vi "Add Thread Configuration.vi"(8 "error in":errorcluster, 10 "configuration":T14, 11 "thread":T1={"core"={"processor"=-2, "priority offset"=0}, "component settings"=[], "transfer groups"=[]}) -> (0 "error out":errorcluster, 3 "thread out":T1={"core"={"processor"=-2, "priority offset"=0}, "component settings"=[], "transfer groups"=[]})   [LabVIEW 2020, in "DSF UDP Configuration API.lvlib"]
uses:
  DSF UDP Configuration API.lvlib
  Built/Plugins/Windows/Components/UDP.lvlibp/Configuration/Thread/Thread Settings.ctl
  <vilib>/addons/VeriStand Custom Device Scripting APIs/Data Sharing Framework/DSF Core.lvlibp/Typedefs/DSF Engine Plugin Thread Configuration.ctl
  <vilib>/addons/VeriStand Custom Device Scripting APIs/Data Sharing Framework/DSF Core.lvlibp/Typedefs/Core Thread Configuration.ctl
  <vilib>/addons/VeriStand Custom Device Scripting APIs/Data Sharing Framework/DSF Core.lvlibp/Typedefs/DSF Settings Info.ctl
  <vilib>/addons/VeriStand Custom Device Scripting APIs/Data Sharing Framework/DSF Core.lvlibp/Typedefs/DSF Engine Transfer Group Configuration.ctl
  <vilib>/addons/VeriStand Custom Device Scripting APIs/Data Sharing Framework/DSF Core.lvlibp/Typedefs/Core Group Configuration.ctl
  <vilib>/addons/VeriStand Custom Device Scripting APIs/Data Sharing Framework/DSF Core.lvlibp/Typedefs/DSF Direction.ctl
  <vilib>/addons/VeriStand Custom Device Scripting APIs/Data Sharing Framework/DSF Core.lvlibp/Typedefs/DSF Timing Info.ctl
  <vilib>/addons/VeriStand Custom Device Scripting APIs/Data Sharing Framework/DSF Core.lvlibp/Typedefs/DSF Timeout Behavior.ctl
  <vilib>/addons/VeriStand Custom Device Scripting APIs/Data Sharing Framework/DSF Core.lvlibp/Typedefs/DSF Engine Transfer Configuration.ctl
  <vilib>/addons/VeriStand Custom Device Scripting APIs/Data Sharing Framework/DSF Core.lvlibp/Typedefs/Core Transfer Configuration.ctl
  <vilib>/addons/VeriStand Custom Device Scripting APIs/Data Sharing Framework/DSF Core.lvlibp/Typedefs/DSF Engine Channel Configuration.ctl
  <vilib>/addons/VeriStand Custom Device Scripting APIs/Data Sharing Framework/DSF Core.lvlibp/Typedefs/Core Channel Configuration.ctl
  <vilib>/addons/VeriStand Custom Device Scripting APIs/Data Sharing Framework/DSF Core.lvlibp/Typedefs/DSF Data Type.ctl
  fab8a0ae-df1d-4f1f-ba96-0da676de6823.vi
  <vilib>/addons/VeriStand Custom Device Scripting APIs/Data Sharing Framework/DSF Core.lvlibp
  Built/Plugins/Windows/Components/UDP.lvlibp/Configuration/Thread/UDP Thread Configuration.lvclass
  <vilib>/addons/VeriStand Custom Device Scripting APIs/Data Sharing Framework/DSF Core.lvlibp/Classes/Configuration/Core/Thread/Thread Configuration.lvclass
  <vilib>/addons/VeriStand Custom Device Scripting APIs/Data Sharing Framework/DSF Core.lvlibp/Classes/Configuration/Core/Group/Group Configuration.lvclass
  <vilib>/addons/VeriStand Custom Device Scripting APIs/Data Sharing Framework/DSF Core.lvlibp/Classes/Configuration/Core/Transfer/Transfer Configuration.lvclass
  <vilib>/addons/VeriStand Custom Device Scripting APIs/Data Sharing Framework/DSF Core.lvlibp/Classes/Configuration/Core/Channel/Channel Configuration.lvclass
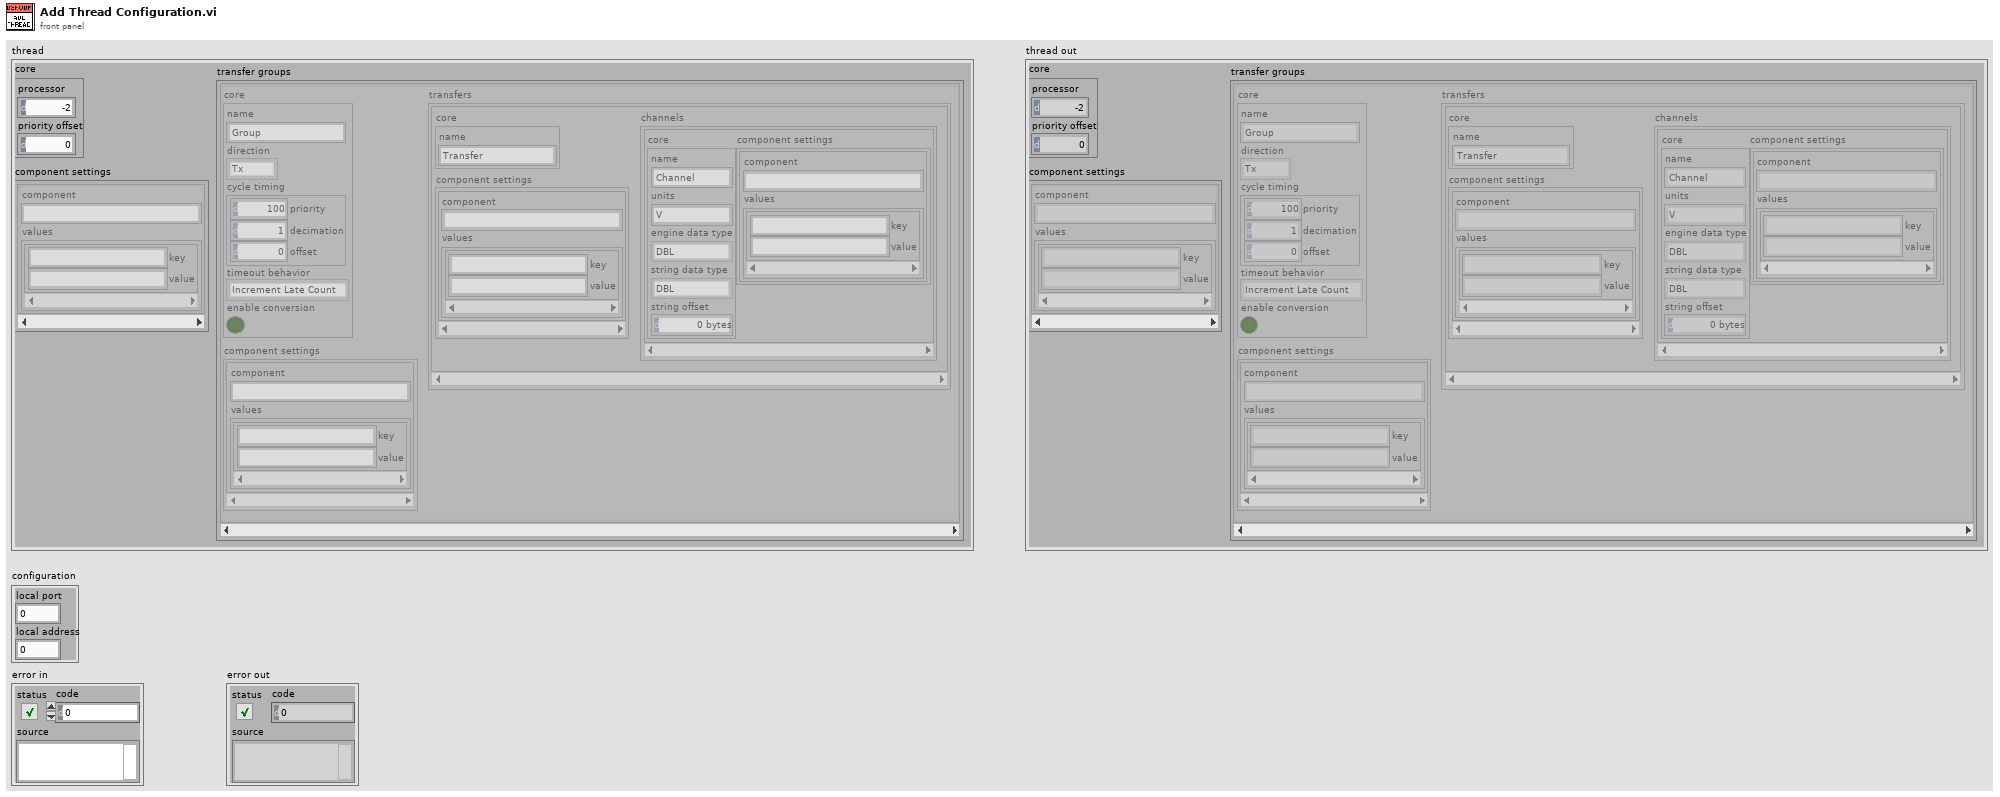
[diagram p1: front panel]
types:
  T1 = typedef "DSF Core.lvlibp/DSF Engine Plugin Thread Configuration.ctl" = cluster{"core":T2, "component settings":T3[], "transfer groups":T4[]}
  T2 = typedef "DSF Core.lvlibp/Thread Configuration.lvclass/Core Thread Configuration.ctl" = cluster{"processor":i32, "priority offset":i16}
  T3 = typedef "DSF Core.lvlibp/DSF Settings Info.ctl" = cluster{"component":string, "values":cluster{"key":string, "value":string}[]}
  T4 = typedef "DSF Core.lvlibp/DSF Engine Transfer Group Configuration.ctl" = cluster{"core":T5, "component settings":T3[], "transfers":T9[]}
  T5 = typedef "DSF Core.lvlibp/Group Configuration.lvclass/Core Group Configuration.ctl" = cluster{"name":string, "direction":T6, "cycle timing":T7, "timeout behavior":T8, "enable conversion":bool}
  T6 = typedef "DSF Core.lvlibp/DSF Direction.ctl" = enum8{"Tx", "Rx"}
  T7 = typedef "DSF Core.lvlibp/DSF Timing Info.ctl" = cluster{"priority":u64, "decimation":u64, "offset":u64}
  T8 = typedef "DSF Core.lvlibp/DSF Timeout Behavior.ctl" = enum8{"Increment Late Count", "Throw Error"}
  T9 = typedef "DSF Core.lvlibp/DSF Engine Transfer Configuration.ctl" = cluster{"core":T10, "component settings":T3[], "channels":T11[]}
  T10 = typedef "DSF Core.lvlibp/Transfer Configuration.lvclass/Core Transfer Configuration.ctl" = cluster{"name":string}
  T11 = typedef "DSF Core.lvlibp/DSF Engine Channel Configuration.ctl" = cluster{"core":T12, "component settings":T3[]}
  T12 = typedef "DSF Core.lvlibp/Channel Configuration.lvclass/Core Channel Configuration.ctl" = cluster{"name":string, "units":string, "engine data type":T13, "string data type":T13, "string offset":u64}
  T13 = typedef "DSF Core.lvlibp/DSF Data Type.ctl" = enum8{"Bool", "SGL", "DBL", "I8", "I16", "I32", "I64", "U8", "U16", "U32", "U64"}
  T14 = typedef "UDP.lvlibp/UDP Thread Configuration.lvclass/Thread Settings.ctl" = cluster{"local port":u16, "local address":u32}
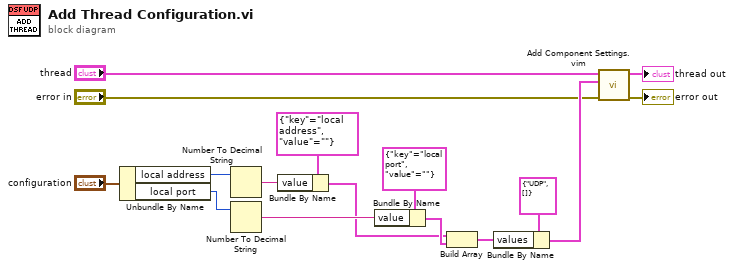
[diagram p0: block diagram]
diagram:
  n1 = Unbundle By Name("configuration") -> ("local address"=w14:u32, "local port"=w13:u16)
  n2 = Number To Decimal String(number=w14) -> (decimal integer string=w11:string)  [unwired: 1 in]
  n3 = Number To Decimal String(number=w13) -> (decimal integer string=w9:string)  [unwired: 1 in]
  n4 = Bundle By Name(cluster=cluster{"key":string, "value":string} {"key"="local address", "value"=""} ("setting"), "value"=w11) -> (w7:cluster{"key":string, "value":string})
  n5 = Bundle By Name(cluster=cluster{"key":string, "value":string} {"key"="local port", "value"=""} ("setting"), "value"=w9) -> (w8:cluster{"key":string, "value":string})
  n6 = Build Array(w7, w8) -> (w6:cluster{"key":string, "value":string}[])
  n7 = Bundle By Name(cluster=T3 {"component"="UDP", "values"=[]} ("component settings"), "values"=w6) -> (w4:T3)
  n8 = call "Add Component Settings.vim"("error in"="error in", "component settings"=w4, "dsf configuration"="thread") -> ("error out"=→"error out":errorcluster, "dsf configuration out"=→"thread out":T1)  [unwired: 7 in]
